vi "Sensor Data (Multiple Readings).vi"(6 "Reading Interval (100)":dbl=100.0, 7 "Sample Count (1)":i32=1, 8 "error in (no error)":errorcluster, 9 "Data Source (0:Kelvin)":u16(ring) items=["Kelvin", "Celsius", "Sensor Units"], 10 "Input (0:A)":u16(ring) items=["A", "B", "C", "D", "D2", "D3", "D4", "D5"], 11 "VISA resource name":refnum<visa-resource-name>) -> (0 "error out":errorcluster, 2 "Sensor Data":dbl[](array[numeric]) format="%#.5f", 3 "VISA resource name out":refnum<visa-resource-name>)   [LabVIEW 2015, in "Lake Shore 350.lvlib"]
doc: "Reads and returns multiple sensor readings from the instrument. Control over interval between readings is also provided."
uses:
  Lake Shore 350.lvlib
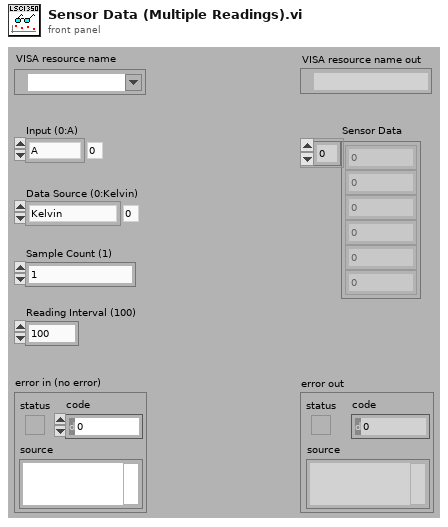
[diagram p1: front panel]
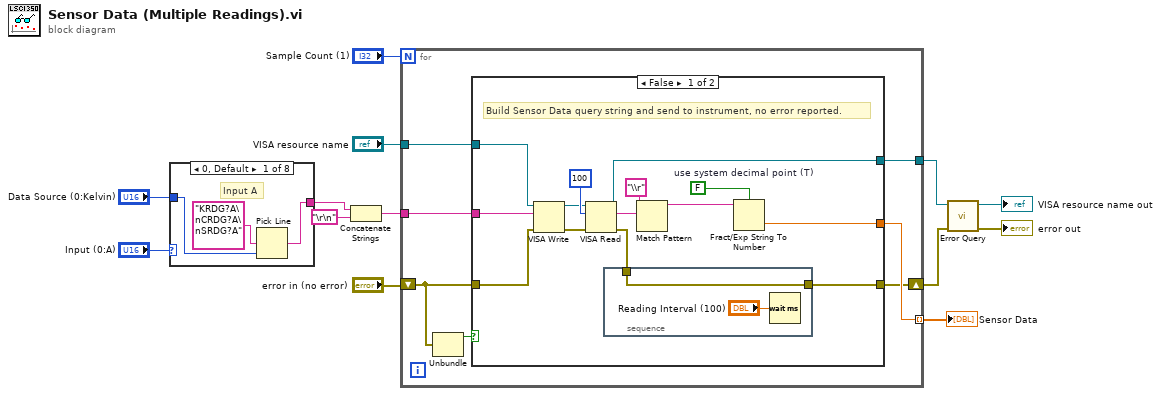
[diagram p0: block diagram]
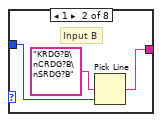
[diagram p2: hidden frame]
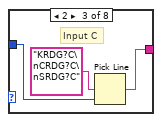
[diagram p3: hidden frame]
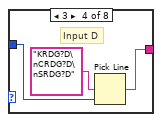
[diagram p4: hidden frame]
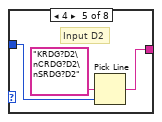
[diagram p5: hidden frame]
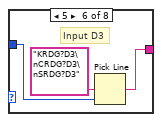
[diagram p6: hidden frame]
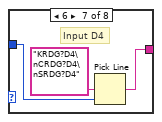
[diagram p7: hidden frame]
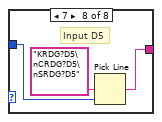
[diagram p8: hidden frame]
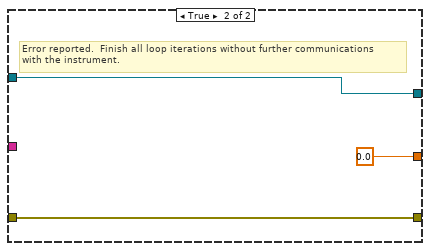
[diagram p9: hidden frame]
diagram:
  n1 = case shown="0, Default" "Input (0:A)" {
    tunnel: "Data Source (0:Kelvin)" -> [w15 w17 w20 w23 w26 w29 w32 w35]
    tunnel: [w14 w18 w21 w24 w27 w30 w33 w36] -> w4
    frame 0, Default {
      # "Input A"
      n2 = Pick Line(multi-line string="KRDG?A\nCRDG?A\nSRDG?A", line index=w15) -> (output string=w14:string)  [unwired: 1 in]
    }
    frame 1 {
      # "Input B"
      n3 = Pick Line(multi-line string="KRDG?B\nCRDG?B\nSRDG?B", line index=w17) -> (output string=w18:string)  [unwired: 1 in]
    }
    frame 2 {
      # "Input C"
      n4 = Pick Line(multi-line string="KRDG?C\nCRDG?C\nSRDG?C", line index=w20) -> (output string=w21:string)  [unwired: 1 in]
    }
    frame 3 {
      # "Input D"
      n5 = Pick Line(multi-line string="KRDG?D\nCRDG?D\nSRDG?D", line index=w23) -> (output string=w24:string)  [unwired: 1 in]
    }
    frame 4 {
      # "Input D2"
      n6 = Pick Line(multi-line string="KRDG?D2\nCRDG?D2\nSRDG?D2", line index=w26) -> (output string=w27:string)  [unwired: 1 in]
    }
    frame 5 {
      # "Input D3"
      n7 = Pick Line(multi-line string="KRDG?D3\nCRDG?D3\nSRDG?D3", line index=w29) -> (output string=w30:string)  [unwired: 1 in]
    }
    frame 6 {
      # "Input D4"
      n8 = Pick Line(multi-line string="KRDG?D4\nCRDG?D4\nSRDG?D4", line index=w32) -> (output string=w33:string)  [unwired: 1 in]
    }
    frame 7 {
      # "Input D5"
      n9 = Pick Line(multi-line string="KRDG?D5\nCRDG?D5\nSRDG?D5", line index=w35) -> (output string=w36:string)  [unwired: 1 in]
    }
  }
  n10 = Concatenate Strings(w4, "\r\n") -> (w3:string)
  n11 = for {
    N: "Sample Count (1)" -> [_]
    tunnel: "VISA resource name" -> [w44]
    tunnel: [w43] -> w10
    tunnel: w3 -> [w42]
    tunnel: [w41] -> w8 mode=indexing
    shift-right: [w40] -> w6
    shift-left: "error in (no error)" -> [w39]
    n12 = Unbundle(w39) -> ("status"=w38:bool)  [unwired: 2 out]
    n13 = case shown="False" w38 {
      tunnel: w44 -> [w58 w63]
      tunnel: [w57 w63] -> w43
      tunnel: w42 -> [w49 _]
      tunnel: [w48 0.0] -> w41
      tunnel: w39 -> [w47 w62]
      tunnel: [w45 w62] -> w40
      frame False {
        w51 = FALSE  # use system decimal point (T)
        # "Build Sensor Data query string and send to instrument, no error reported."
        n14 = VISA Write(VISA resource name=w58, write buffer=w49, error in (no error)=w47) -> (VISA resource name out=w53:refnum<visa-resource-name>, error out=w52:errorcluster)  [unwired: 1 out]
        n15 = VISA Read(VISA resource name=w53, byte count=100, error in (no error)=w52) -> (VISA resource name out=w57:refnum<visa-resource-name>, read buffer=w55:string, error out=w46:errorcluster)  [unwired: 1 out]
        n16 = stacked-sequence {
          tunnel: w46 -> [w59]
          tunnel: [w59] -> w45
          frame #0 {
            n17 = Wait (ms)(milliseconds to wait="Reading Interval (100)") -> ()  [unwired: 1 out]
          }
        }
        n18 = Match Pattern(string=w55, regular expression="\\r") -> (before substring=w50:string)  [unwired: 1 in, 3 out]
        n19 = Fract/Exp String To Number(use system decimal point (T)=w51, string=w50) -> (number=w48:dbl)  [unwired: 2 in, 1 out]
      }
      frame True {
        # "Error reported.  Finish all loop iterations without further communications\nwith the instrument."
      }
    }
  }
  "Sensor Data" <- w8
  n20 = call "Error Query.vi"("error in (no error)"=w6, "VISA resource name"=w10) -> ("error out"=→"error out":errorcluster, "VISA resource name out"=→"VISA resource name out":refnum<visa-resource-name>)  [unwired: 7 in, 1 out]
